vi "CheckLibraryDeployed.vi"(8 "error in (no error)":errorcluster, 10 "Container Name":string, 11 "Target IP":string) -> (0 "error out":errorcluster, 3 "needsDeploy":bool)   [LabVIEW 2013]
uses:
  <resource>/objmgr/ni.var.rc
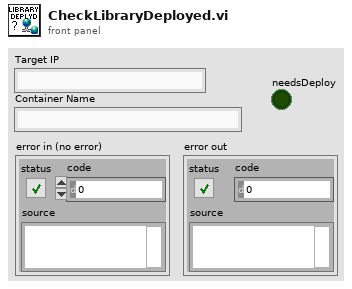
[diagram p1: front panel]
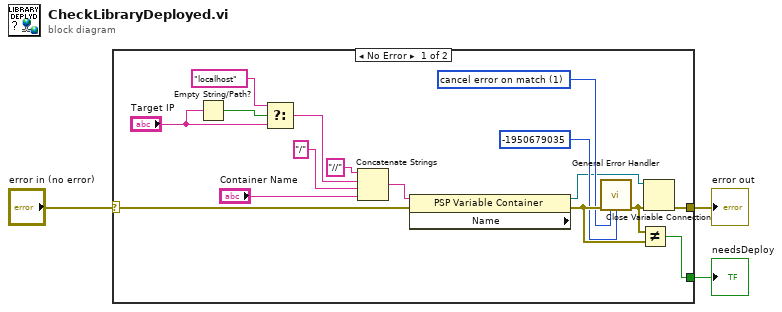
[diagram p0: block diagram]
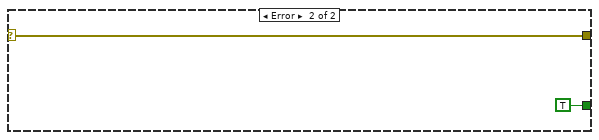
[diagram p2: hidden frame]
diagram:
  n1 = case shown="No Error" "error in (no error)" {
    selector: "error in (no error)" -> [w4 w21]
    tunnel: [w14 TRUE] -> w3
    tunnel: [w5 w21] -> w2
    frame No Error {
      w17 = 1 items=["no exception", "cancel error on match", "set error on match"] ("[exception action] (none:0)")
      n2 = Empty String/Path?(string/path="Target IP") -> (empty?=w7:bool)
      n3 = Select(t="localhost" ("AlarmsEvents:Database Computer"), s=w7, f="Target IP") -> (s? t:f=w9:string)
      n4 = Concatenate Strings("//" ("string"), w9, "/" ("string"), "Container Name") -> (w11:string)
      n5 = property class="PSP Variable Container" props=["Name"](reference=w11, error in=w4) -> (reference out=w16:refnum<k21>, error out=w19:errorcluster)  [unwired: 1 out]
      n6 = call <vilib>:"General Error Handler.vi"("error in (no error)"=w19, "[exception action] (none:0)"=w17, "[exception code]"=-1950679035 ("code")) -> ("error out"=w15:errorcluster)  [unwired: 8 in, 4 out]
      n7 = Not Equal?(x=w15, y=w19) -> (x != y?=w14:bool)
      n8 = Close Variable Connection(8:w15, 11:w16) -> (0:w5:errorcluster)
    }
    frame Error {
    }
  }
  "needsDeploy" <- w3
  "error out" <- w2
